vi "writeToXML.vi"(8 "error in (no error)":errorcluster, 10 "Class Label":string="Declination", 11 "Declination in":refnum<class "Declination.lvclass">) -> (0 "error out":errorcluster, 2 "XML out":string="<Declination>\n  <degreesDec>0</degreesDec>\n  <minutesArc>0</minutesArc>\n  <secondsArc>0</secondsArc>\n</Declination>", 3 "Declination out":refnum<class "Declination.lvclass">)   [LabVIEW 2022 SP3, in "TCSDataDefinitions.lvlib" / "TCSCommand.lvlib" / "TargetConfiguration.lvlib" / "Target.lvlib" / "FixedTarget.lvlib" / "Declination.lvclass"]
uses:
  Declination.lvclass
  <userlib>/Common/UnitsAndXML/FlattenItemWithUnitToXML/FlattenPlaneAngleToXML/PlaneAngleUnit.ctl
  Declination.lvclass/Declination.ctl
  <userlib>/Common/UnitsAndXML/UnitsAndXML.lvlib
  <userlib>/Common/XML/XMLGenerator/XMLGenerator.lvclass
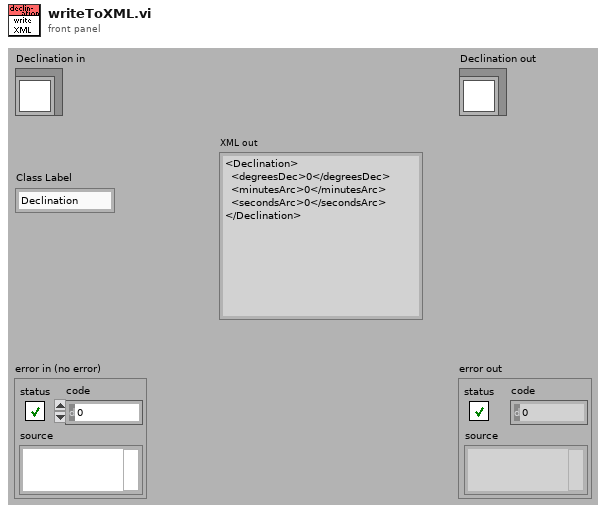
[diagram p1: front panel]
types:
  T1 = typedef "UnitsAndXML.lvlib/PlaneAngleUnit.ctl" = enum16{"rad", "deg", "'", "\""}
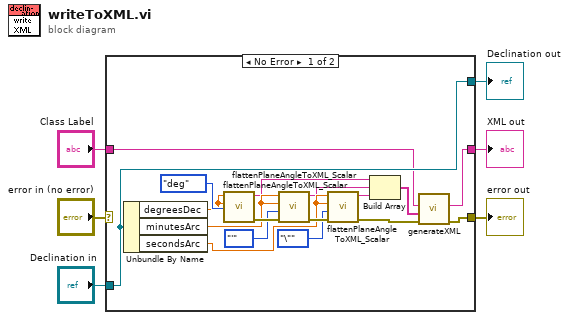
[diagram p0: block diagram]
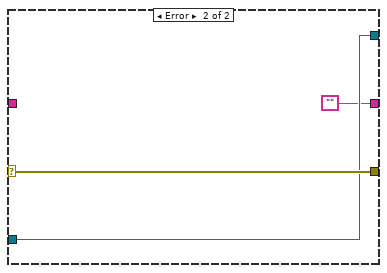
[diagram p2: hidden frame]
diagram:
  n1 = case shown="No Error" "error in (no error)" {
    selector: "error in (no error)" -> [_ w26]
    tunnel: [w9 w26] -> w5
    tunnel: [w15 w25] -> w3
    tunnel: "Declination in" -> [w15 w25]
    tunnel: [w8 ""] -> w2
    tunnel: "Class Label" -> [w7 _]
    frame No Error {
      n2 = Unbundle By Name(w15) -> ("degreesDec"=w18:dbl[unit], "minutesArc"=w17:dbl[unit], "secondsArc"=w16:dbl[unit])
      n3 = call <userlib>:"flattenPlaneAngleToXML_Scalar.vi"("planeAngleUnitInXML"=PlaneAngleUnit."deg", "planeAngleAgain"=w18, "planeAngle"=w18) -> ("error out"=w23:errorcluster, "xmlString"=w14:string)  [unwired: 7 in]
      n4 = call <userlib>:"flattenPlaneAngleToXML_Scalar.vi"("error in (no error)"=w23, "planeAngleUnitInXML"=PlaneAngleUnit."'", "planeAngleAgain"=w17, "planeAngle"=w17) -> ("error out"=w22:errorcluster, "xmlString"=w13:string)  [unwired: 6 in]
      n5 = call <userlib>:"flattenPlaneAngleToXML_Scalar.vi"("error in (no error)"=w22, "planeAngleUnitInXML"=PlaneAngleUnit."\"", "planeAngleAgain"=w16, "planeAngle"=w16) -> ("error out"=w10:errorcluster, "xmlString"=w12:string)  [unwired: 6 in]
      n6 = Build Array(w14, w13, w12) -> (w11:string[])
      n7 = call <userlib>:"generateXML.vi"("error in"=w10, "childrenXML"=w11, "elementName"=w7) -> ("error out"=w9:errorcluster, "XML out"=w8:string)  [unwired: 6 in, 1 out]
    }
    frame Error {
    }
  }
  "error out" <- w5
  "Declination out" <- w3
  "XML out" <- w2
